vi "Histogram.vi"(3 "Error":string, 4 "Histogram":i32[](array[numeric]), 5 "Input Image":T1={"Image ID"=0, "Channel ID"=-1}) -> (0 "Error":string, 1 "Histogram":i32[](array[numeric]), 2 "Input Image":T1={"Image ID"=0, "Channel ID"=-1})   [LabVIEW 2011, in "labvvis.lvlib"]
doc: "Returns an array with 256 elements, where each element in the array contains the number of times pixels equal to the index is encountered in Input Image.\n\nIf you connect an array that does not have 256 elements, this VI will not execute. If you do not connect an array at all, this VI will provide one.\n\nNote that this VI only operates on single-channel images. Thus grey-scale, Red channel, Green channel and so on images are supported. RGBA images are not supported."
uses:
  <userlib>/labvvis/labvvis.lvlib
  <userlib>/labvvis/VVIS Image.ctl
  labvvis.framework
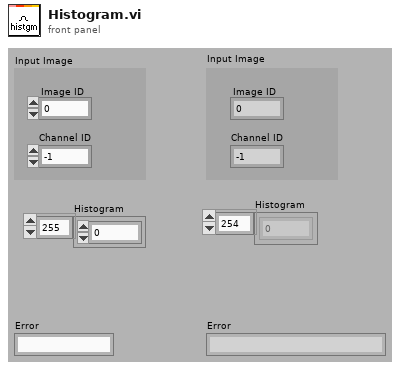
[diagram p1: front panel]
types:
  T1 = typedef "labvvis.lvlib/VVIS Image.ctl" = cluster{"Image ID":i16, "Channel ID":i16}
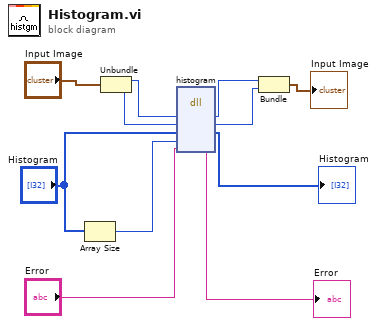
[diagram p0: block diagram]
diagram:
  n1 = Array Size(array="Histogram") -> (size(s)=w9:i32)
  n2 = Unbundle("Input Image") -> ("Image ID"=w10:i16, "Channel ID"=w4:i16)
  n3 = dll-call lib="labvvis.framework" fn="histogram"("src1"=w10, "cid"=w4, "counts"="Histogram", "counts_size"=w9, "Error") -> ("src1"=w3:i16, "cid"=w2:i16, "counts"=→"Histogram":i32[], →"Error":string)  [unwired: 5 in, 2 out]
  n4 = Bundle("src1"=w3, "cid"=w2) -> (→"Input Image":cluster{"src1":i16, "cid":i16})  [unwired: 1 in]
